vi "initialise_scanners.vi"(8 "error in (no error)":errorcluster, 11 "DL090202ScanHead in":refnum<class "ScanHeadDL090202.lvclass">) -> (0 "error out":errorcluster, 3 "DL090202ScanHead out":refnum<class "ScanHeadDL090202.lvclass">)   [LabVIEW 2010, in "ScanHeadDL090202.lvclass"]
uses:
  ScanHeadDL090202.lvclass
  Trajectory/TrajectoryDL091126GenericVoxel/TrajectoryDL091126GenericVoxel/TrajectoryDL091126GenericVoxel.lvclass
  Trajectory/GenericTrajectory/GenericTrajectory/GenericTrajectory.lvclass
  SignalWriter/GenericSignalWriter/GenericSignalWriter/GenericSignalWriter.lvclass
  common/classes/ErrorController/ErrorController/class_data.vi
  common/classes/ErrorController/ErrorController/ErrorController.lvclass
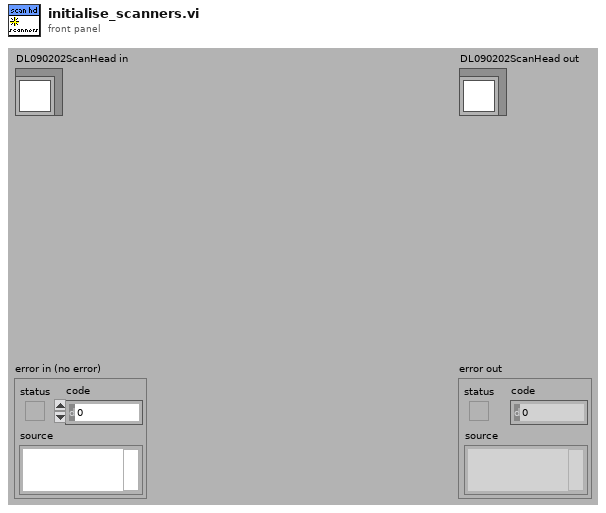
[diagram p1: front panel]
types:
  T1 = typedef "counter_settings_cluster.ctl" = cluster{"offset cycles":i32, "high cycles":i32, "low cycles":i32}
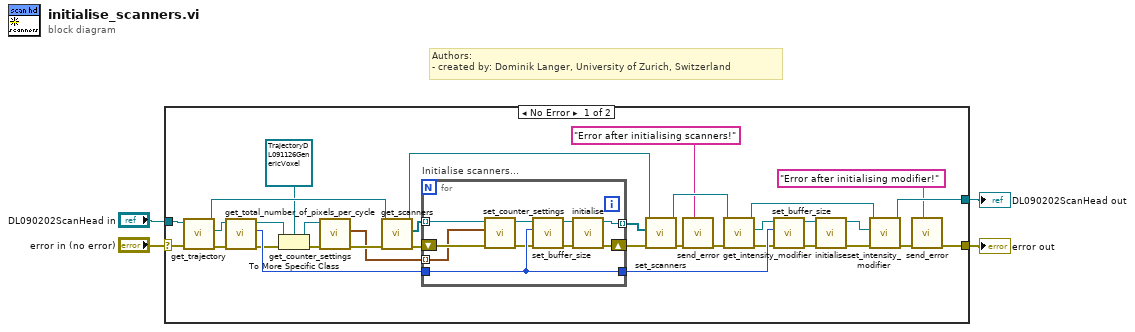
[diagram p0: block diagram]
diagram:
  # "Authors: \n- created by: Dominik Langer, University of Zurich, Switzerland"
  n1 = case shown="No Error" "error in (no error)" {
    selector: "error in (no error)" -> [w24 w50]
    tunnel: [w7 w50] -> w3
    tunnel: [w22 w49] -> w1
    tunnel: "DL090202ScanHead in" -> [w23 w49]
    frame No Error {
      n2 = call-dynamic "get_trajectory.vi"("error in (no error)"=w24, "GenericScanHead.lvclass in"=w23) -> ("error out"=w25:errorcluster, "trajectory"=w26:refnum<class "GenericTrajectory.lvclass">, "GenericScanHead.lvclass out"=w21:refnum<class "ScanHeadDL090202.lvclass">)  [unwired: 7 out]
      n3 = call-dynamic "get_total_number_of_pixels_per_cycle.vi"("error in (no error)"=w25, "GenericTrajectory in"=w26) -> ("error out"=w17:errorcluster, "total number of pixels per cycle"=w20:i32, "GenericTrajectory out"=w15:refnum<class "GenericTrajectory.lvclass">)  [unwired: 7 out]
      n4 = To More Specific Class(target class=refnum<class "TrajectoryDL091126GenericVoxel.lvclass"> refnum ("TrajectoryDL091126GenericVoxel.lvclass"), reference=w15, error in=w17) -> (specific class reference=w14:refnum<class "TrajectoryDL091126GenericVoxel.lvclass">, error out=w16:errorcluster)
      n5 = call-dynamic "get_counter_settings.vi"("error in (no error)"=w16, "TrajectoryDL091126GenericVoxel in"=w14) -> ("error out"=w19:errorcluster, "counter settings"=w13:T1[])  [unwired: 7 in, 1 out]
      n6 = call-dynamic "get_scanners.vi"("error in (no error)"=w19, "DL090202ScanHead.lvclass in"=w21) -> ("error out"=w37:errorcluster, "scanners"=w36:refnum<class "GenericSignalWriter.lvclass">[], "DL090202ScanHead.lvclass out"=w30:refnum<class "ScanHeadDL090202.lvclass">)  [unwired: 7 out]
      n7 = for "Initialise scanners..." {
        shift-right: [w44] -> w35
        shift-left: w37 -> [w43]
        tunnel: w36 -> [w40] mode=indexing
        tunnel: [w48] -> w33 mode=indexing
        tunnel: w20 -> [w45]
        tunnel: [w45] -> w38
        tunnel: w13 -> [w39] mode=indexing
        n8 = call-dynamic "set_counter_settings.vi"("error in (no error)"=w43, "counter"=w39, "GenericSignalWriter in"=w40) -> ("error out"=w42:errorcluster, "GenericSignalWriter out"=w41:refnum<class "GenericSignalWriter.lvclass">)  [unwired: 7 in]
        n9 = call-dynamic "set_buffer_size.vi"("error in (no error)"=w42, "buffer size (samples)"=w45, "GenericWriteSignals.lvclass in"=w41) -> ("error out"=w46:errorcluster, "GenericWriteSignals.lvclass out"=w47:refnum<class "GenericSignalWriter.lvclass">)  [unwired: 7 out]
        n10 = call-dynamic "initialise.vi"("error in (no error)"=w46, "GenericPlugin in"=w47) -> ("error out"=w44:errorcluster, "GenericPlugin out"=w48:refnum<class "GenericSignalWriter.lvclass">)  [unwired: 8 out]
      }
      n11 = call-dynamic "set_scanners.vi"("error in (no error)"=w35, "scanners"=w33, "DL090202ScanHead.lvclass in"=w30) -> ("error out"=w10:errorcluster, "DL090202ScanHead.lvclass out"=w32:refnum<class "ScanHeadDL090202.lvclass">)  [unwired: 7 out]
      n12 = call "send_error.vi"("additional message"="Error after initialising scanners!", "error in (no error)"=w10) -> ("error out"=w9:errorcluster)  [unwired: 9 in]
      n13 = call-dynamic "get_intensity_modifier.vi"("error in (no error)"=w9, "DL090202ScanHead.lvclass in"=w32) -> ("error out"=w34:errorcluster, "write signals"=w31:refnum<class "GenericSignalWriter.lvclass">, "DL090202ScanHead.lvclass out"=w28:refnum<class "ScanHeadDL090202.lvclass">)  [unwired: 7 out]
      n14 = call-dynamic "set_buffer_size.vi"("error in (no error)"=w34, "buffer size (samples)"=w38, "GenericWriteSignals.lvclass in"=w31) -> ("error out"=w12:errorcluster, "GenericWriteSignals.lvclass out"=w11:refnum<class "GenericSignalWriter.lvclass">)  [unwired: 7 out]
      n15 = call-dynamic "initialise.vi"("error in (no error)"=w12, "GenericPlugin in"=w11) -> ("error out"=w29:errorcluster, "GenericPlugin out"=w27:refnum<class "GenericSignalWriter.lvclass">)  [unwired: 8 out]
      n16 = call-dynamic "set_intensity_modifier.vi"("error in (no error)"=w29, "write signals"=w27, "DL090202ScanHead.lvclass in"=w28) -> ("error out"=w8:errorcluster, "DL090202ScanHead.lvclass out"=w22:refnum<class "ScanHeadDL090202.lvclass">)  [unwired: 7 out]
      n17 = call "send_error.vi"("additional message"="Error after initialising modifier!", "error in (no error)"=w8) -> ("error out"=w7:errorcluster)  [unwired: 9 in]
    }
    frame Error {
    }
  }
  "error out" <- w3
  "DL090202ScanHead out" <- w1
